vi "niLvFpga_Abort_cRIO-9039 (Sync).vi"(0 "session in":u32, 11 "error in":errorcluster) -> (4 "session out":u32, 15 "error out":errorcluster)   [LabVIEW 2017]
uses:
  NiFpgaLv.dll
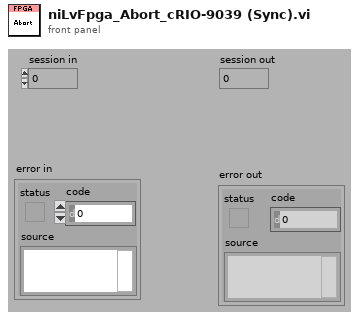
[diagram p1: front panel]
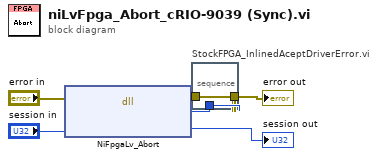
[diagram p0: block diagram]
diagram:
  n1 = dll-call lib="NiFpgaLv.*" fn="NiFpgaLv_Abort" label="niLvFpgaAbort"(error in="error in", "sessionID"="session in") -> (error out=w3:errorcluster, "status"=w1:i32, "sessionID"=→"session out":u32)  [unwired: 2 in, 1 out]
  n2 = stacked-sequence "StockFPGA_InlinedAceptDriverError.vi" {
    tunnel: w3 -> [w7]
    tunnel: w1 -> [w9]
    tunnel: [w8] -> w2
    frame #0 {
      n3 = case shown="Default" w9 {
        selector: w9 -> [_ w11]
        tunnel: [w10 w13] -> w8
        tunnel: w7 -> [w10 w14]
        frame 0 {
        }
        frame Default {
          n4 = Greater Than 0?(x=w11) -> (x > 0?=w12:bool)
          n5 = call <vilib>:"Error Cluster From Error Code.vi"("is warning? (False)"=w12, "error in (no error)"=w14, "error code (0)"=w11) -> ("error out"=w13:errorcluster)  [unwired: 6 in]
        }
      }
    }
  }
  "error out" <- w2
